vi "TrajectoryState_Equals.vi"(9 "Other TRAJ_STATE":T1={"TimeSeconds"=0.0, "Velocity"=0.0, "Acceleration"=0.0, "POSE"={"TRANSLATION"={"X"=0.0, "Y"=0.0}, "ROTATION"={"VALUE"=0.0, "COS"=1.0, "SIN"=0.0}}, "Curvature"=0.0} {"POSE"."ROTATION"."SIN" format="%13.4f"; "POSE"."ROTATION"."COS" format="%13.4f"; "POSE"."ROTATION"."VALUE" format="%13.4f"; "POSE"."TRANSLATION"."Y" format="%14.3f"; "POSE"."TRANSLATION"."X" format="%14.3f"}, 11 "TRAJ_STATE":T1={"TimeSeconds"=0.0, "Velocity"=0.0, "Acceleration"=0.0, "POSE"={"TRANSLATION"={"X"=0.0, "Y"=0.0}, "ROTATION"={"VALUE"=0.0, "COS"=1.0, "SIN"=0.0}}, "Curvature"=0.0} {"POSE"."ROTATION"."SIN" format="%13.4f"; "POSE"."ROTATION"."COS" format="%13.4f"; "POSE"."ROTATION"."VALUE" format="%13.4f"; "POSE"."TRANSLATION"."Y" format="%14.3f"; "POSE"."TRANSLATION"."X" format="%14.3f"}) -> (3 "Equals":bool)   [LabVIEW 2019, in "Trajectory_Library.lvlib"]
doc: "Determines if two Trajectory States are equal\n \nParameters:\n - TrajState - TrajectoryState data structure\n - Other TrajState - Other TrajectoryState data structure\n \nReturns:\n - Equals - boolean indicating if the states are equal."
uses:
  Trajectory_Library.lvlib
  TRANSLATION2D.ctl
  ROTATION2D.ctl
  POSE2D.ctl
  TRAJ_STATE.ctl
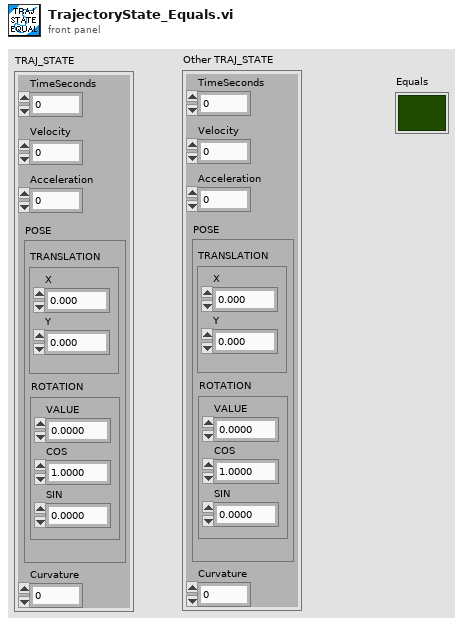
[diagram p1: front panel]
types:
  T1 = typedef "Trajectory_Library.lvlib/TRAJ_STATE.ctl" = cluster{"TimeSeconds":dbl, "Velocity":dbl, "Acceleration":dbl, "POSE":T2, "Curvature":dbl}
  T2 = typedef "Trajectory_Library.lvlib/POSE2D.ctl" = cluster{"TRANSLATION":T3, "ROTATION":T4}
  T3 = typedef "Trajectory_Library.lvlib/TRANSLATION2D.ctl" = cluster{"X":dbl, "Y":dbl}
  T4 = typedef "Trajectory_Library.lvlib/ROTATION2D.ctl" = cluster{"VALUE":dbl, "COS":dbl, "SIN":dbl}
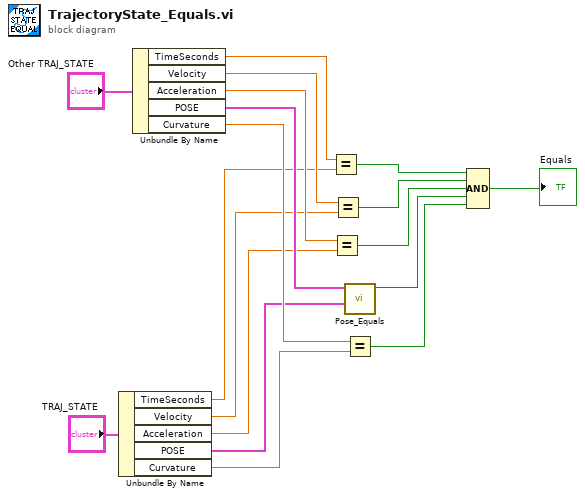
[diagram p0: block diagram]
diagram:
  n1 = Unbundle By Name("TRAJ_STATE") -> ("TimeSeconds"=w7:dbl, "Velocity"=w8:dbl, "Acceleration"=w9:dbl, "POSE"=w10:T2, "Curvature"=w11:dbl)
  n2 = Unbundle By Name("Other TRAJ_STATE") -> ("TimeSeconds"=w16:dbl, "Velocity"=w15:dbl, "Acceleration"=w14:dbl, "POSE"=w13:T2, "Curvature"=w12:dbl)
  n3 = Equal?(x=w16, y=w7) -> (x = y?=w6:bool)
  n4 = Equal?(x=w14, y=w9) -> (x = y?=w4:bool)
  n5 = Equal?(x=w15, y=w8) -> (x = y?=w5:bool)
  n6 = call "Pose_Equals.vi"("other POSE"=w10, "in POSE"=w13) -> ("Equals"=w3:bool)  [unwired: 9 in]
  n7 = Equal?(x=w12, y=w11) -> (x = y?=w2:bool)
  n8 = Compound Arithmetic op=AND(w6, w5, w4, w3, w2) -> (→"Equals":bool)
